vi "Create Message Queues.vi"(8 "error in (no error)":errorcluster) -> (0 "error out":errorcluster, 3 "Message Queues":T1)   [LabVIEW 2017, in "Vibratome.lvlib"]
uses:
  Vibratome.lvlib
  Message Queues.ctl
  Support VIs/Message Queue/Message.ctl
  Support VIs/Message Queue/Enqueue Message (Single).vi
  Support VIs/Message Queue/Message Queue.lvlib
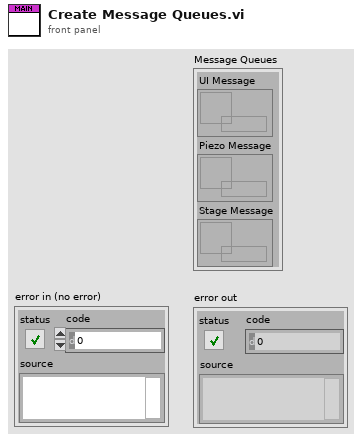
[diagram p1: front panel]
types:
  T1 = typedef "Vibratome.lvlib/Message Queues.ctl" = cluster{"UI Message":refnum<queue>, "Piezo Message":refnum<queue>, "Stage Message":refnum<queue>}
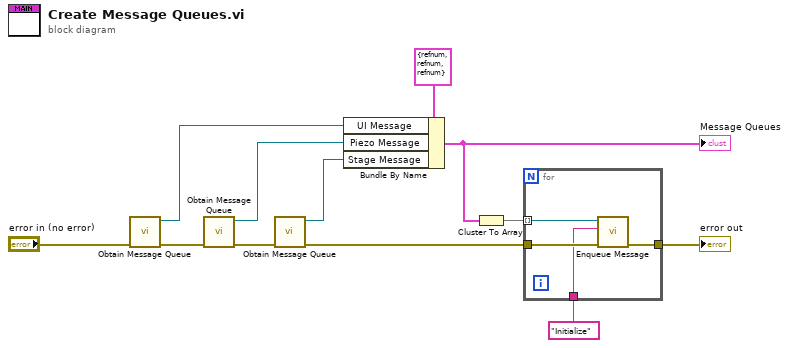
[diagram p0: block diagram]
diagram:
  n1 = call "Obtain Message Queue.vi"("error in (no error)"="error in (no error)") -> ("error out"=w12:errorcluster, "Message Queue out"=w7:refnum<queue>)  [unwired: 9 in]
  n2 = call "Obtain Message Queue.vi"("error in (no error)"=w12) -> ("error out"=w9:errorcluster, "Message Queue out"=w11:refnum<queue>)  [unwired: 9 in]
  n3 = call "Obtain Message Queue.vi"("error in (no error)"=w9) -> ("error out"=w4:errorcluster, "Message Queue out"=w8:refnum<queue>)  [unwired: 9 in]
  n4 = Bundle By Name(cluster=T1 {"UI Message"=refnum, "Piezo Message"=refnum, "Stage Message"=refnum} ("Queues"), "UI Message"=w7, "Piezo Message"=w11, "Stage Message"=w8) -> (w6:T1)
  "Message Queues" <- w6
  n5 = Cluster To Array(cluster=w6) -> (array=w5:refnum<queue>[])
  n6 = for {
    tunnel: w5 -> [w16] mode=indexing
    tunnel: w4 -> [w15]
    tunnel: "Initialize" ("State") -> [w14]
    tunnel: [w13] -> w2
    n7 = call-poly "Enqueue Message.vi"("error in (no error)"=w15, "State"=w14, "Message Queue in"=w16) -> ("error out"=w13:errorcluster)  [unwired: 7 in, 1 out]
  }
  "error out" <- w2
